vi "Run All.vi"(8 "Error In":errorcluster) -> (0 "Error Out":errorcluster)   [LabVIEW 2017, in "Tests.lvlib" / "KnownHosts.lvlib"]
uses:
  KnownHosts.lvlib
  <vilib>/addons/_JKI Toolkits/Caraya/classes/Test/Test.lvclass
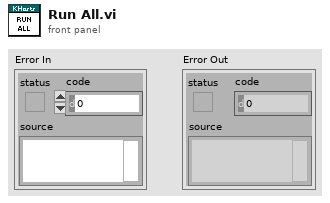
[diagram p1: front panel]
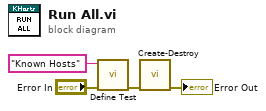
[diagram p0: block diagram]
diagram:
  n1 = call <vilib>:"Define Test.vi"("error in (no error)"="Error In", "Label (VI Title)"="Known Hosts") -> ("error out"=w2:errorcluster)  [unwired: 9 in]
  n2 = call "Create-Destroy.vi"("Error In"=w2) -> ("Error Out"=→"Error Out":errorcluster)  [unwired: 10 in]
